vi "Solenoid_Loop_ACT.vi"() -> ()   [LabVIEW 2016, in "WC_Drive.lvlib"]
uses:
  WC_Drive.lvlib
  Globals/Global_STOP.vi
  System Templates/TemplateActuator/Global_ACT Write_Data Out.vi
  System Templates/TemplateActuator/TemplateActuator.lvlib
  <vilib>/Rock Robotics/WPI/Solenoid/WPI_SolenoidChannel.ctl
  Globals/Global_CMD_Gear.vi
  <vilib>/Rock Robotics/WPI/Solenoid/WPI_SolenoidOpenDouble.vi
  <vilib>/Rock Robotics/WPI/Solenoid/WPI_SolenoidSetEnum.vi
panel:
  out "Output Data":dbl
  out "Input Data":dbl
  out "Cycle Time (S)":dbl format="%.3g"
  in  "Target Time(ms)":u32=50
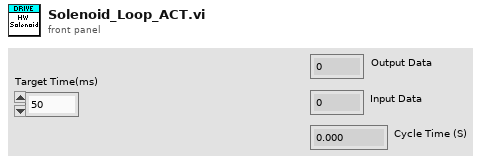
[diagram p1: front panel]
types:
  T1 = typedef "WPI_SolenoidChannel.ctl" = enum8{"Solenoid 0", "Solenoid 1", "Solenoid 2", "Solenoid 3", "Solenoid 4", "Solenoid 5", "Solenoid 6", "Solenoid 7", "Invalid"}
  T2 = typedef "WPI_SolenoidDevRef.ctl" = cluster{"DevStatus":errorcluster, "Pneumatics Control Module":u8, "Forward Solenoid Channel":T1, "Reverse Solenoid Channel":T1}
  T3 = cluster{"SolenoidDevRef":T2, "Solenoid Out (T) In(F)":bool, "Target Time(ms)":u32, "Current Time":timestamp, "Previous Time":timestamp, "Cycle Time (S)":dbl}
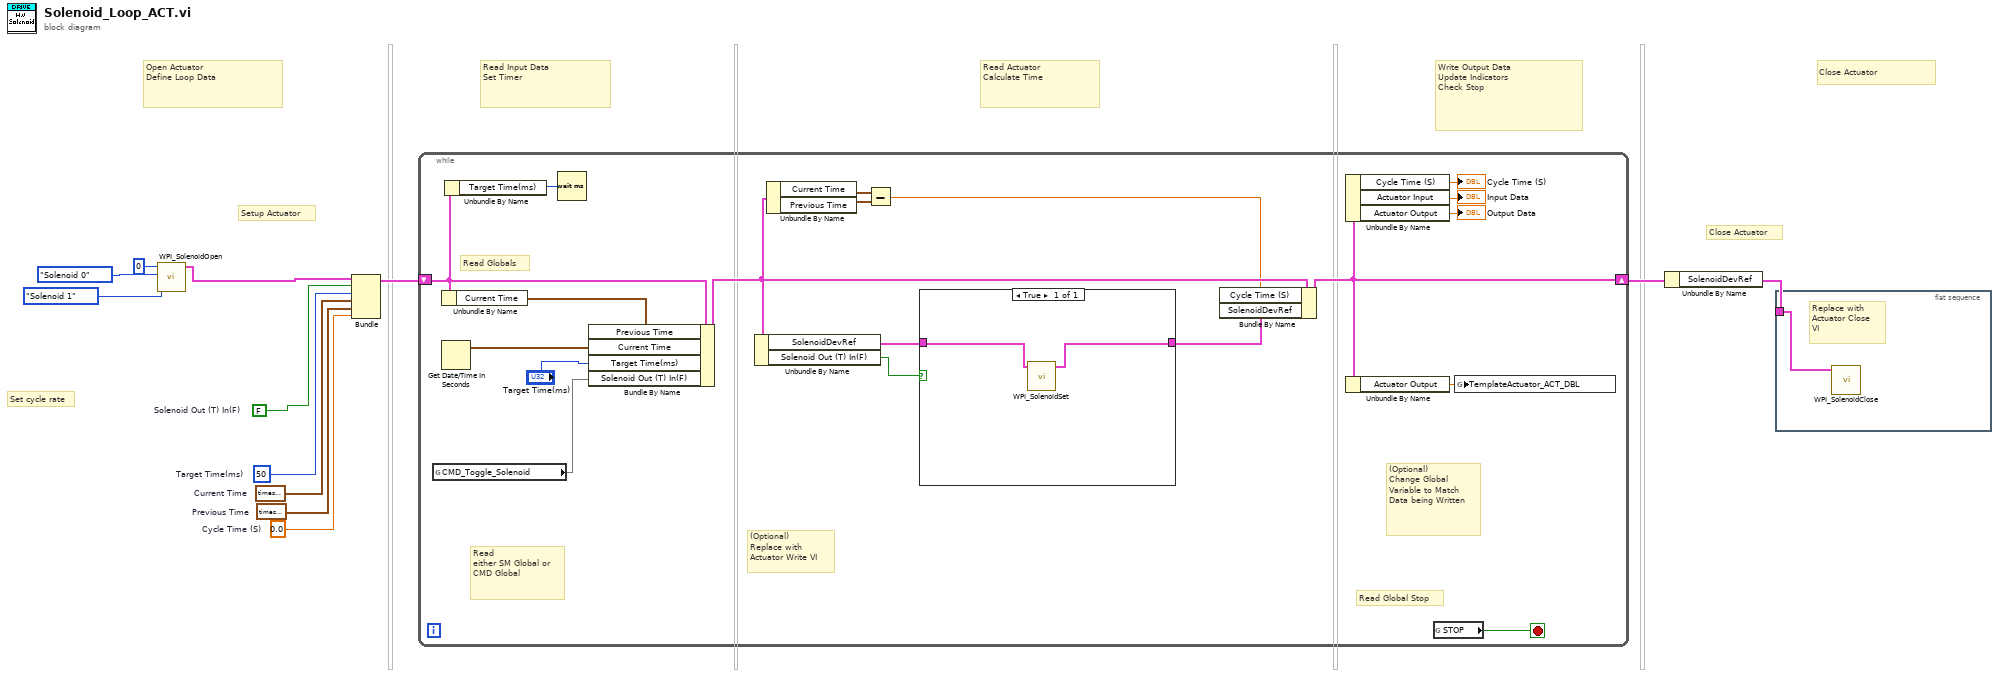
[diagram p0: block diagram]
diagram:
  w4 = FALSE  # Solenoid Out (T) In(F)
  w5 = 0.0  # Cycle Time (S)
  w12 = timestamp(0 s since 1904-01-01)  # Previous Time
  w11 = timestamp(0 s since 1904-01-01)  # Current Time
  w10 = u32 50  # Target Time(ms)
  # "Close Actuator"
  # "Write Output Data\nUpdate Indicators\nCheck Stop"
  # "Read Actuator\nCalculate Time"
  # "Read Input Data\nSet Timer"
  # "Open Actuator\nDefine Loop Data"
  # "Set cycle rate"
  # "Close Actuator"
  # "Setup Actuator"
  n1 = call-poly <vilib>:"WPI_SolenoidOpen.vi"("Reverse Solenoid Channel"=WPI_SolenoidChannel."Solenoid 1", "Forward Solenoid Channel"=WPI_SolenoidChannel."Solenoid 0", "Pneumatics Control Module (0)"=u8 0) -> ("SolenoidDevRef"=w7:T2)  [unwired: 7 in, 1 out]
  n2 = Bundle("SolenoidDevRef"=w7, "Solenoid Out (T) In(F)"=w4, "Target Time(ms)"=w10, "Current Time"=w11, "Previous Time"=w12, "Cycle Time (S)"=w5) -> (w8:T3)  [unwired: 1 in]
  n3 = while {
    shift-right: [w20] -> w6
    shift-left: w8 -> [w22]
    stop <- w31 stop-if-true
    # "(Optional)\nReplace with\nActuator Write VI"
    # "(Optional)\nChange Global\nVariable to Match\nData being Written"
    # "Read\neither SM Global or CMD Global"
    # "Read Globals"
    # "Read Global Stop"
    n4 = global read "Global_CMD_Gear.vi" "CMD_Toggle_Solenoid"() -> (w14)
    n5 = Unbundle By Name(w22) -> ("Current Time"=w27:timestamp)
    n6 = Get Date/Time In Seconds() -> (seconds since 1Jan1904=w28:timestamp)
    n7 = Unbundle By Name(w22) -> ("Target Time(ms)"=w21:u32)
    n8 = Wait (ms)(milliseconds to wait=w21) -> ()  [unwired: 1 out]
    n9 = Bundle By Name(cluster=w22, "Previous Time"=w27, "Current Time"=w28, "Target Time(ms)"="Target Time(ms)", "Solenoid Out (T) In(F)"=w14) -> (w23:T3)
    n10 = Unbundle By Name(w23) -> ("SolenoidDevRef"=w30:T2, "Solenoid Out (T) In(F)"=w13:bool)
    n11 = Unbundle By Name(w23) -> ("Current Time"=w26:timestamp, "Previous Time"=w25:timestamp)
    n12 = Subtract(x=w26, y=w25) -> (x-y=w16:dbl)
    n13 = case shown="True" w13 {
      tunnel: w30 -> [w33]
      tunnel: [w32] -> w29
      frame True {
        n14 = call-poly <vilib>:"WPI_SolenoidSet.vi"("SolenoidDevRef"=w33) -> ("SolenoidDevRef"=w32:T2)  [unwired: 9 in, 1 out]
      }
    }
    n15 = Bundle By Name(cluster=w23, "Cycle Time (S)"=w16, "SolenoidDevRef"=w29) -> (w20:T3)
    n16 = Unbundle By Name(w20) -> ("Cycle Time (S)"=→"Cycle Time (S)":dbl, "Actuator Input"=→"Input Data":dbl, "Actuator Output"=→"Output Data":dbl)
    n17 = Unbundle By Name(w20) -> ("Actuator Output"=w15:dbl)
    n18 = global read "Global_STOP.vi" "STOP"() -> (w31:bool)
    n19 = global write "Global_ACT Write_Data Out.vi" "TemplateActuator_ACT_DBL"(w15) -> ()
  }
  n20 = Unbundle By Name(w6) -> ("SolenoidDevRef"=w9:T2)
  n21 = flat-sequence {
    tunnel: w9 -> [w34]
    frame #0 {
      # "Replace with \nActuator Close\nVI"
      n22 = call <vilib>:"WPI_SolenoidClose.vi"("SolenoidDevRef"=w34) -> ()  [unwired: 10 in, 1 out]
    }
  }
